vi "Remove From SubPanel.vi"(8 "error in (no error)":errorcluster, 11 "ViewableActor in":refnum<class "ViewableActor.lvclass">) -> (0 "error out":errorcluster, 3 "ViewableActor out":refnum<class "ViewableActor.lvclass">)   [LabVIEW 2020, in "ViewableActor.lvlib" / "ViewableActor.lvclass"]
uses:
  ViewableActor.lvclass
  ViewableActor.lvclass/ViewableActor.ctl
  Read SubPanel Ref.vi
  Write SubPanel Ref.vi
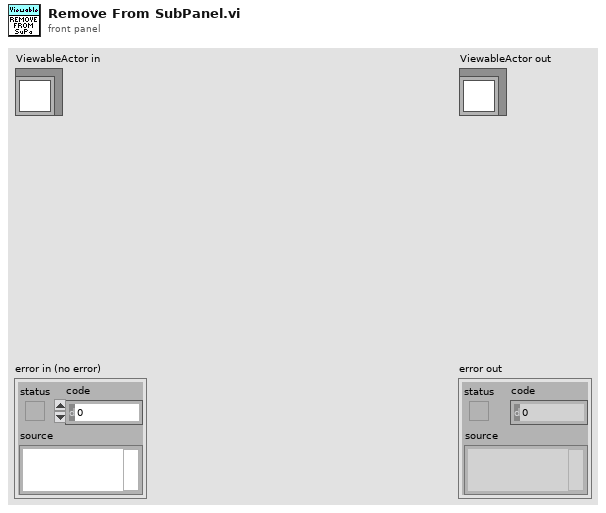
[diagram p1: front panel]
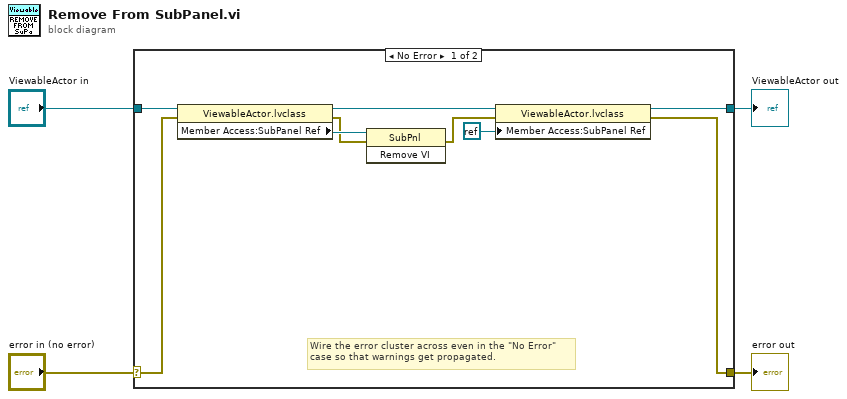
[diagram p0: block diagram]
diagram:
  n1 = case shown="No Error" "error in (no error)" {
    selector: "error in (no error)" -> [w6 w15]
    tunnel: [w5 w15] -> w3
    tunnel: [w11 w14] -> w1
    tunnel: "ViewableActor in" -> [w13 w14]
    frame No Error {
      # "Wire the error cluster across even in the \"No Error\"\ncase so that warnings get propagated."
      n2 = property class="ViewableActor.lvclass"(reference=w13, error in=w6) -> (reference out=w12:refnum<class "ViewableActor.lvclass">, error out=w8:errorcluster, "Member Access:SubPanel Ref"=w9:refnum<vi>)
      n3 = invoke class="SubPnl" method="Remove VI"(reference=w9, error in=w8) -> (error out=w7:errorcluster)  [unwired: 1 in, 2 out]
      n4 = property class="ViewableActor.lvclass"(reference=w12, error in=w7, "Member Access:SubPanel Ref"=refnum<k0> refnum) -> (reference out=w11:refnum<class "ViewableActor.lvclass">, error out=w5:errorcluster)
    }
    frame Error {
    }
  }
  "error out" <- w3
  "ViewableActor out" <- w1
